vi "2022_day07.vi"() -> ()   [LabVIEW 2021]
uses:
  3baf8011-b907-4a24-9a6c-8a8b08bbcfa0.vi
  <vilib>/Comparison/Less/Less Functor/Less Functor.lvclass
panel:
  out "Task 2":i32
  out "Total Used Space":i32
  out "Task 1":i32
  in  "Switch":bool caption="Ex. Data  vs.  User Data"
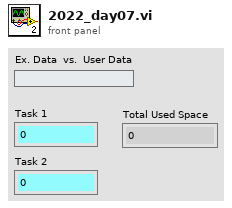
[diagram p1: front panel]
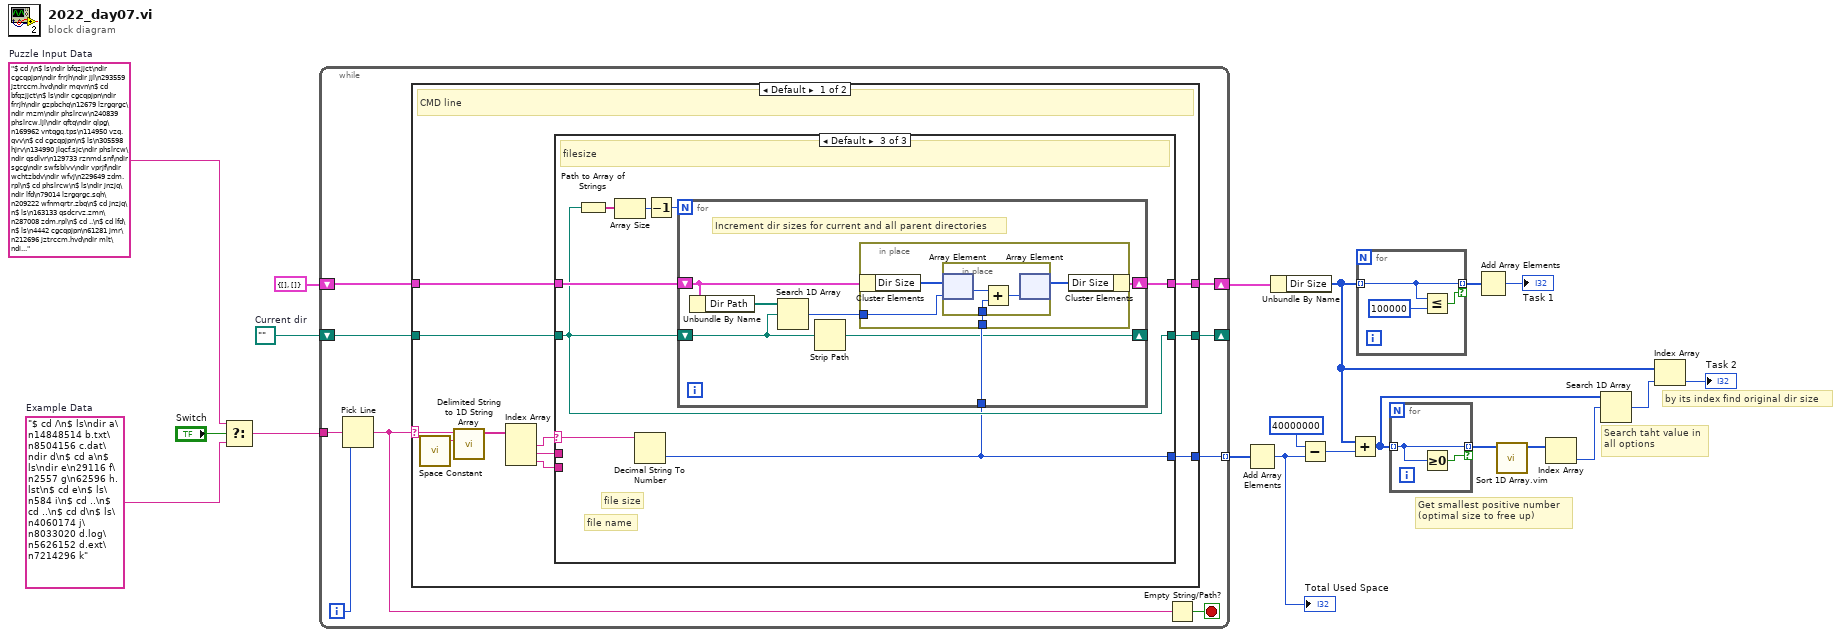
[diagram p0: block diagram]
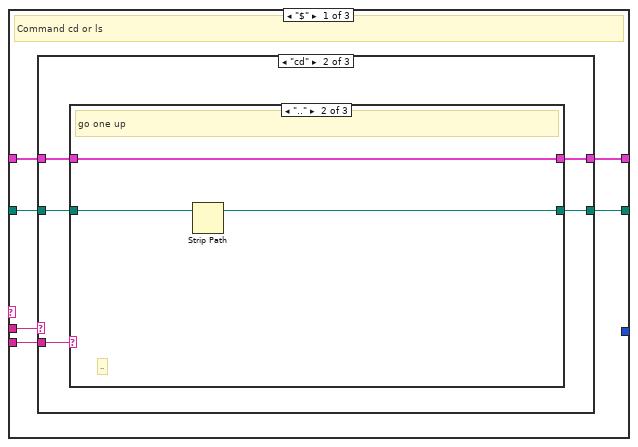
[diagram p2: hidden frame]
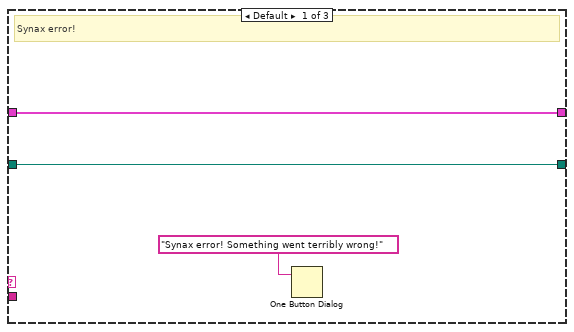
[diagram p3: hidden frame]
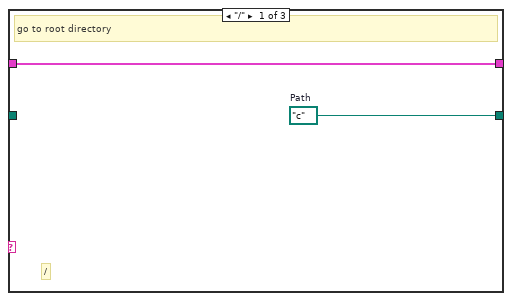
[diagram p4: hidden frame]
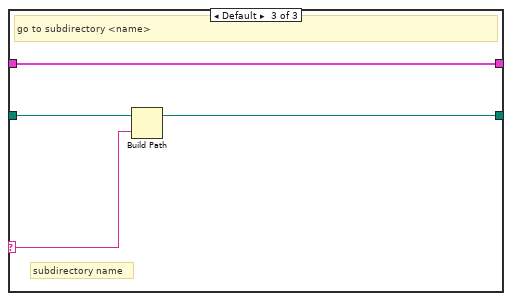
[diagram p5: hidden frame]
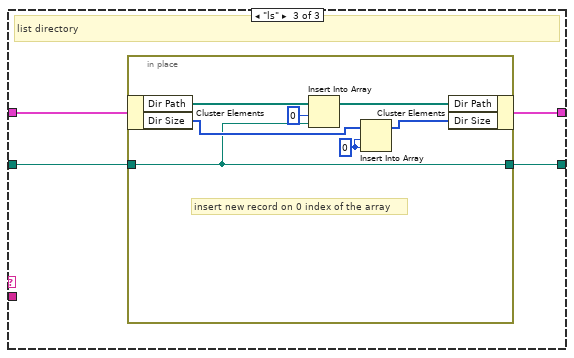
[diagram p6: hidden frame]
diagram:
  w15 = path ""  # Current dir
  w19 = "$ cd /\n$ ls\ndir bfqzjjct\ndir cgcqpjpn\ndir frrjh\ndir jjl\n293559 jztrccm.hvd\ndir mqvn\n$ cd bfqzjjct\n$ ls\ndir cgcqpjpn\ndir frrjh\ndir gzpbchq\n12679 lzrgqrgc\ndir mzm\ndir phslrcw\n240839 phslrcw.ljl\ndir qftq\ndir qlpg\n169962 vntqgq.tps\n114950 vzq.qvv\n$ cd cgcqpjpn\n$ ls\n305598 hjrv\n134990 jlqcf.sjc\ndir phslrcw\ndir qsdlvr\n129733 rznmd.snf\ndir sgcg\ndir swfsblvv\ndir vprjf\ndir wchtzbdv\ndir wfvj\n229649 zdm.rpl\n$ cd phslrcw\n$ ls\ndir jnzjq\ndir lfd\n79014 lzrgqrgc.sqh\n209222 wfnmqrtr.zbq\n$ cd jnzjq\n$ ls\n163133 qsdcrvz.zmn\n287008 zdm.rpl\n$ cd ..\n$ cd lfd\n$ ls\n4442 cgcqpjpn\n61281 jmr\n212696 jztrccm.hvd\ndir mlt\ndir qsdlvr\n$ cd mlt\n$ ls\n183050 zdm.rpl\n$ cd ..\n$ cd qsdlvr\n$ ls\ndir nzjfwdt\ndir qsdlvr\n$ cd nzjfwdt\n$ ls\n49044 jdqz.bqd\n$ cd ..\n$ cd qsdlvr\n$ ls\n13838 fpfmhq.rbp\n$ cd ..\n$ cd ..\n$ cd ..\n$ cd ..\n$ cd qsdlvr\n$ ls\n167042 jdqz.bqd\n132914 lzrgqrgc\n$ cd ..\n$ cd sgcg\n$ ls\ndir bjwzfr\n111567 jdqz.bqd\n33253 jztrccm.hvd\n75760 qsdlvr\n$ cd bjwzfr\n$ ls\n268763 npjd.glz\ndir phslrcw\n121486 vbfsrwf.mbc\ndir vtwtmnvl\n$ cd phslrcw\n$ ls\n114641 cgsrlq\n235130 npjd.glz\n$ cd ..\n$ cd vtwtmnvl\n$ ls\n7771 hnrpgsn\n290862 rtrljz.vbf\n220102 rztn.vqq\n$ cd ..\n$ cd ..\n$ cd ..\n$ cd swfsblvv\n$ ls\n231282 vclmcf.vpq\n16727 vjhmb.ftn\n$ cd ..\n$ cd vprjf\n$ ls\ndir fppsf\n56173 npjd.glz\ndir phslrcw\ndir pwjdcdff\ndir qsdlvr\ndir qvh\ndir sbmtlz\n$ cd fppsf\n$ ls\ndir hltnf\ndir qrmggjs\ndir qsdlvr\n$ cd hltnf\n$ ls\n201448 npjd.glz\n23616 zdm.rpl\n$ cd ..\n$ cd qrmggjs\n$ ls\ndir blhwqwd\ndir szf\n$ cd blhwqwd\n$ ls\n142887 vzq.qvv\n$ cd ..\n$ cd szf\n$ ls\n225491 tvsf.tpv\n$ cd ..\n$ cd ..\n$ cd qsdlvr\n$ ls\n92209 brmrwznr\ndir frrjh\n212979 qsdlvr.bwh\ndir vpvnb\n$ cd frrjh\n$ ls\n143811 qvwmpj.gnc\n$ cd ..\n$ cd vpvnb\n$ ls\ndir wwsw\n$ cd wwsw\n$ ls\n13671 qsdlvr\n$ cd ..\n$ cd ..\n$ cd ..\n$ cd ..\n$ cd phslrcw\n$ ls\ndir bpfhc\ndir fjvgwbj\n127950 hjngrw.rtr\n37045 lfpjb.ftz\ndir qsn\n$ cd bpfhc\n$ ls\n232351 frrjh.szf\n14824 jztrccm.hvd\n162270 vzq.qvv\n$ cd ..\n$ cd fjvgwbj\n$ ls\ndir cgcqpjpn\n4290 jrfsmghw.vqr\ndir lqnpdd\n$ cd cgcqpjpn\n$ ls\n208104 btrcq.vpn\n149676 bwvp.jlf\n76056 gvvrvqdf.zdc\n272686 pqhtjpv\ndir zjntbw\n$ cd zjntbw\n$ ls\n140092 jdqz.bqd\n$ cd ..\n$ cd ..\n$ cd lqnpdd\n$ ls\ndir brf\n197899 jdqz.bqd\ndir phslrcw\n236823 qcvgnlv.ngn\ndir szrfcwtw\n88974 vzq.qvv\n$ cd brf\n$ ls\n112059 jdqz.bqd\n217412 vzq.qvv\n$ cd ..\n$ cd phslrcw\n$ ls\n84285 jnzf\n282660 zdm.rpl\n$ cd ..\n$ cd szrfcwtw\n$ ls\n84415 gcp\n163787 wffb.wbq\n$ cd ..\n$ cd ..\n$ cd ..\n$ cd qsn\n$ ls\n139676 zdm.rpl\n$ cd ..\n$ cd ..\n$ cd pwjdcdff\n$ ls\ndir cgcqpjpn\n54163 lzrgqrgc\ndir qsdlvr\n51246 qsdlvr.cmq\n5082 rvmv.tqj\n112712 vzq.qvv\n$ cd cgcqpjpn\n$ ls\n92895 dmf.bsv\ndir lhqzc\n$ cd lhqzc\n$ ls\n13443 hwlsmmjn.wpj\n232141 tlsn\n$ cd ..\n$ cd ..\n$ cd qsdlvr\n$ ls\n216144 dghbz.lnl\n241311 jztrccm.hvd\n$ cd ..\n$ cd ..\n$ cd qsdlvr\n$ ls\n109764 qsdlvr.tbj\n$ cd ..\n$ cd qvh\n$ ls\ndir frrjh\n51428 hdtmm.zzl\n$ cd frrjh\n$ ls\n271661 brff.mgp\n$ cd ..\n$ cd ..\n$ cd sbmtlz\n$ ls\n277255 jztrccm.hvd\n$ cd ..\n$ cd ..\n$ cd wchtzbdv\n$ ls\n198310 cgcqpjpn\n300478 fcfvgpdr.lzv\n145860 jdqz.bqd\n20145 mggg\n$ cd ..\n$ cd wfvj\n$ ls\n270522 phslrcw.mwt\n213919 tczvr\n19226 zdm.rpl\n$ cd ..\n$ cd ..\n$ cd frrjh\n$ ls\ndir cgcqpjpn\n246391 hnc.bzl\ndir lzrgqrgc\ndir mnrbzwr\n239337 npjd.glz\ndir qsdlvr\n$ cd cgcqpjpn\n$ ls\n2423 pflhrgjg.gch\n$ cd ..\n$ cd lzrgqrgc\n$ ls\n265708 vzq.qvv\n107406 zwnjb\n$ cd ..\n$ cd mnrbzwr\n$ ls\n287289 jgs.bdb\n$ cd ..\n$ cd qsdlvr\n$ ls\ndir qsdlvr\n$ cd qsdlvr\n$ ls\n71204 gnfz\n$ cd ..\n$ cd ..\n$ cd ..\n$ cd gzpbchq\n$ ls\ndir cmqgph\ndir fwf\n146975 jztrccm.hvd\n284515 lzrgqrgc.qsf\n27455 qbsbvscc\n$ cd cmqgph\n$ ls\n177740 zdm.rpl\n$ cd ..\n$ cd fwf\n$ ls\n210658 dnmvdgwn.wzt\n22013 rqcspw.qmf\n244013 zdm.rpl\n$ cd ..\n$ cd ..\n$ cd mzm\n$ ls\n262805 gnfsbdcd.tvp\n$ cd ..\n$ cd phslrcw\n$ ls\n74949 wncqjc.tzd\n$ cd ..\n$ cd qftq\n$ ls\ndir jrds\n$ cd jrds\n$ ls\ndir dvht\ndir qsdlvr\n$ cd dvht\n$ ls\n57354 phslrcw\n57174 qsdlvr.ftm\n$ cd ..\n$ cd qsdlvr\n$ ls\n132030 fbsmfspp\n$ cd ..\n$ cd ..\n$ cd ..\n$ cd qlpg\n$ ls\ndir cgcqpjpn\ndir frrjh\ndir jjsfmg\n186178 jmvcvw\ndir qgjhlnmf\n100234 qltp.vdr\ndir tbwt\ndir vjjvfbdw\ndir wjz\n162428 zlbnsg\n$ cd cgcqpjpn\n$ ls\ndir gvmgcftp\ndir hsgvgc\ndir nps\ndir phslrcw\ndir scdglb\n$ cd gvmgcftp\n$ ls\n31869 dsddwbbp\ndir fbsrjgzj\n53280 tzn.fvp\n$ cd fbsrjgzj\n$ ls\n89267 qsdlvr.lhs\n$ cd ..\n$ cd ..\n$ cd hsgvgc\n$ ls\ndir lzrgqrgc\n210774 wpspf.vrd\n$ cd lzrgqrgc\n$ ls\n289086 gfhwwslq.tlz\n$ cd ..\n$ cd ..\n$ cd nps\n$ ls\n74713 fnqzcr\ndir srjvfq\n94736 wbrcn.nng\ndir wmddln\ndir zsgnrmcc\n$ cd srjvfq\n$ ls\ndir grqft\ndir pjnjlf\n254618 wmfnmfrc.wng\n$ cd grqft\n$ ls\n3742 zmpzwh.nvz\n$ cd ..\n$ cd pjnjlf\n$ ls\ndir mlrsrs\n$ cd mlrsrs\n$ ls\n167149 jztrccm.hvd\n$ cd ..\n$ cd ..\n$ cd ..\n$ cd wmddln\n$ ls\n222831 cgcqpjpn.dcv\n140188 gsvngqp\n174466 sfngrqgj.gvz\n$ cd ..\n$ cd zsgnrmcc\n$ ls\n143043 vzq.qvv\n$ cd ..\n$ cd ..\n$ cd phslrcw\n$ ls\ndir cdfsrvnc\n103523 hzsjc\n239089 jvwdjbq\n229835 npjd.glz\n189778 wwcccwmb.bdp\n$ cd cdfsrvnc\n$ ls\ndir vzsvcnlz\n$ cd vzsvcnlz\n$ ls\ndir wwn\n$ cd wwn\n$ ls\n60279 frngbwm.wwf\n$ cd ..\n$ cd ..\n$ cd ..\n$ cd ..\n$ cd scdglb\n$ ls\n176557 vzq.qvv\n$ cd ..\n$ cd ..\n$ cd frrjh\n$ ls\n130811 jdqz.bqd\n$ cd ..\n$ cd jjsfmg\n$ ls\ndir nffq\n22842 vzt.nwh\n$ cd nffq\n$ ls\ndir wmq\n$ cd wmq\n$ ls\n196322 jztrccm.hvd\n$ cd ..\n$ cd ..\n$ cd ..\n$ cd qgjhlnmf\n$ ls\ndir jhqqjt\ndir phslrcw\n246296 pzvmcq\n219308 tlhqgtcl.twb\ndir vfgb\n300258 zdm.rpl\n221663 zsqh.dph\n$ cd jhqqjt\n$ ls\n90068 fctpjdlm.ggg\ndir frrjh\ndir ngmzbqb\ndir phslrcw\n64341 qsdlvr.pnq\ndir vlgpcg\n$ cd frrjh\n$ ls\n49247 qrrhdhld.sjr\n$ cd ..\n$ cd ngmzbqb\n$ ls\n247800 cgcqpjpn.wgv\n$ cd ..\n$ cd phslrcw\n$ ls\ndir qsdlvr\ndir vjrrrm\n$ cd qsdlvr\n$ ls\n255302 ddvc\n182817 dzd.trp\n$ cd ..\n$ cd vjrrrm\n$ ls\n38983 hjbsqd.pdl\n$ cd ..\n$ cd ..\n$ cd vlgpcg\n$ ls\ndir frrjh\n83387 jztrccm.hvd\n$ cd frrjh\n$ ls\ndir rmlc\n$ cd rmlc\n$ ls\n273584 jztrccm.hvd\n$ cd ..\n$ cd ..\n$ cd ..\n$ cd ..\n$ cd phslrcw\n$ ls\n96286 jztrccm.hvd\n224425 npjd.glz\n$ cd ..\n$ cd vfgb\n$ ls\ndir fgl\ndir fllsgwjt\ndir frrjh\ndir qsdlvr\n$ cd fgl\n$ ls\n61972 lzrgqrgc.qrs\n$ cd ..\n$ cd fllsgwjt\n$ ls\ndir fqchdcpd\n214477 zcr.spz\n$ cd fqchdcpd\n$ ls\n156000 jccqlw.twl\n$ cd ..\n$ cd ..\n$ cd frrjh\n$ ls\n210987 zdm.rpl\n$ cd ..\n$ cd qsdlvr\n$ ls\ndir phslrcw\ndir znnsfvz\n$ cd phslrcw\n$ ls\n214655 ddw\n$ cd ..\n$ cd znnsfvz\n$ ls\n126028 zpq.bgs\n$ cd ..\n$ cd ..\n$ cd ..\n$ cd ..\n$ cd tbwt\n$ ls\ndir ltjjhr\n$ cd ltjjhr\n$ ls\n158069 vplwrz.rzp\n$ cd ..\n$ cd ..\n$ cd vjjvfbdw\n$ ls\n277114 fmndb.rth\n241524 frrjh\n212152 frrjh.dlq\n61370 jztrccm.hvd\ndir srvqm\n237264 znt\n$ cd srvqm\n$ ls\ndir fbzmddc\n61958 jdqz.bqd\ndir phslrcw\n173063 vwvmhwzn.tvg\n$ cd fbzmddc\n$ ls\ndir ccvtbpzw\n201647 lzrgqrgc.sjs\n192449 rhfgcgz\n224557 sbcpcbpd\n$ cd ccvtbpzw\n$ ls\ndir phslrcw\ndir prpllzcn\n$ cd phslrcw\n$ ls\n290780 lbl.qmm\n$ cd ..\n$ cd prpllzcn\n$ ls\n242024 bhq\n118347 frrjh.tsz\ndir hcqs\n$ cd hcqs\n$ ls\n104706 csnllvcf\n270940 npjd.glz\n$ cd ..\n$ cd ..\n$ cd ..\n$ cd ..\n$ cd phslrcw\n$ ls\n244909 czfjsrns.fdm\ndir frrjh\n68252 lzrgqrgc\n146640 npjd.glz\n290259 pbzpthgs.bgf\n99657 rmfpfmd\ndir zllf\n$ cd frrjh\n$ ls\ndir cgcqpjpn\n65295 jdqz.bqd\ndir phslrcw\n$ cd cgcqpjpn\n$ ls\ndir mwfwrd\n$ cd mwfwrd\n$ ls\n26481 sngtgc\ndir zfzddl\n$ cd zfzddl\n$ ls\n47854 fzfdrmbb.ngm\n$ cd ..\n$ cd ..\n$ cd ..\n$ cd phslrcw\n$ ls\n251021 fwfpd.vrt\n230149 fwjznjtz\n140480 gbsmhj\n112221 lzrgqrgc.gcr\n139564 npjd.glz\ndir pvmvm\ndir tpzr\n$ cd pvmvm\n$ ls\n73785 tnbgmgt.wqg\n$ cd ..\n$ cd tpzr\n$ ls\n16759 tmcmp\n$ cd ..\n$ cd ..\n$ cd ..\n$ cd zllf\n$ ls\n281402 dzrsnzh.smb\n$ cd ..\n$ cd ..\n$ cd ..\n$ cd ..\n$ cd wjz\n$ ls\n266826 cgcqpjpn.spr\ndir frvbfjj\n111126 jdqz.bqd\n257951 pbn.gdc\ndir vjs\ndir zrnvnb\n$ cd frvbfjj\n$ ls\n257181 glfdplrm\n$ cd ..\n$ cd vjs\n$ ls\ndir jmpbwhtj\n159996 lzrgqrgc.zcb\n192135 phw\ndir tdfz\ndir wtm\n$ cd jmpbwhtj\n$ ls\ndir fln\ndir frrjh\ndir nrtcmj\n$ cd fln\n$ ls\n284574 frrjh.scb\n$ cd ..\n$ cd frrjh\n$ ls\n10020 npjd.glz\n295395 vzq.qvv\n$ cd ..\n$ cd nrtcmj\n$ ls\ndir htvm\n$ cd htvm\n$ ls\ndir lwh\n$ cd lwh\n$ ls\n162494 npjd.glz\n$ cd ..\n$ cd ..\n$ cd ..\n$ cd ..\n$ cd tdfz\n$ ls\ndir gtvlbhhw\ndir hvssbj\ndir phslrcw\n$ cd gtvlbhhw\n$ ls\n172627 sjvcfz\ndir tfnhsrc\n76460 vvgcv\n$ cd tfnhsrc\n$ ls\ndir hjrjmrwc\n$ cd hjrjmrwc\n$ ls\n41459 jztrccm.hvd\n$ cd ..\n$ cd ..\n$ cd ..\n$ cd hvssbj\n$ ls\n64052 phslrcw\n$ cd ..\n$ cd phslrcw\n$ ls\ndir wtdpf\ndir zctdqwbc\n$ cd wtdpf\n$ ls\n75802 jztrccm.hvd\n$ cd ..\n$ cd zctdqwbc\n$ ls\n127648 vqzcf.wbl\n$ cd ..\n$ cd ..\n$ cd ..\n$ cd wtm\n$ ls\n265433 jztrccm.hvd\n20952 mplbrzlp\n123701 nwr.tjg\n58492 qsdlvr.qzq\n$ cd ..\n$ cd ..\n$ cd zrnvnb\n$ ls\n228205 ghllsc.fqn\n$ cd ..\n$ cd ..\n$ cd ..\n$ cd ..\n$ cd cgcqpjpn\n$ ls\ndir cmnsbsqp\ndir hzsn\n221975 jdqz.bqd\n177439 jztrccm.hvd\ndir mqjrcw\ndir tdp\n211065 zdm.rpl\n$ cd cmnsbsqp\n$ ls\n282903 qzlc\n$ cd ..\n$ cd hzsn\n$ ls\n221345 wtdnp.grd\n$ cd ..\n$ cd mqjrcw\n$ ls\n156244 gznmpr.dlr\n45213 hdb.fjb\n202993 pdt\ndir znvdz\n$ cd znvdz\n$ ls\n183973 jztrccm.hvd\n$ cd ..\n$ cd ..\n$ cd tdp\n$ ls\n68564 nmntwl\n259117 vzq.qvv\n$ cd ..\n$ cd ..\n$ cd frrjh\n$ ls\n276034 lzrgqrgc.fgq\ndir psqczq\ndir qsdlvr\ndir snrw\n$ cd psqczq\n$ ls\n158415 jdqz.bqd\n127684 lhctqnnz.hgn\n123191 phslrcw.prl\ndir wrftp\n$ cd wrftp\n$ ls\n234327 qdbbl.czd\n$ cd ..\n$ cd ..\n$ cd qsdlvr\n$ ls\n179591 chbns.sqf\n88327 jdqz.bqd\ndir mrf\n$ cd mrf\n$ ls\n229849 phslrcw.rdr\n$ cd ..\n$ cd ..\n$ cd snrw\n$ ls\ndir cbvr\ndir lbbrtc\n134786 lzrgqrgc.vrt\n131987 vzq.qvv\n$ cd cbvr\n$ ls\n120330 htmgqj.nbq\n162963 lzrgqrgc.rwq\n$ cd ..\n$ cd lbbrtc\n$ ls\ndir tnqdj\n$ cd tnqdj\n$ ls\n72261 lhqnwns.nhj\n235520 qsdlvr.dtr\n$ cd ..\n$ cd ..\n$ cd ..\n$ cd ..\n$ cd jjl\n$ ls\ndir fcfpptw\ndir frrjh\ndir gmdwgs\n221258 jdqz.bqd\ndir lzrgqrgc\ndir mwnmjjj\n297139 smjtpl.zzs\n$ cd fcfpptw\n$ ls\n167264 frrjh\n101587 hsmhhc.lvb\n$ cd ..\n$ cd frrjh\n$ ls\n268280 jztrccm.hvd\n127939 nbqgvd\n247875 nmnrsqq\ndir phslrcw\ndir rmgwbq\n288264 znrrdmw\n$ cd phslrcw\n$ ls\ndir cgcqpjpn\ndir nbwjw\n$ cd cgcqpjpn\n$ ls\n249503 phslrcw.dmf\n$ cd ..\n$ cd nbwjw\n$ ls\ndir phslrcw\n$ cd phslrcw\n$ ls\n193336 sqpgwtgp.fpb\n$ cd ..\n$ cd ..\n$ cd ..\n$ cd rmgwbq\n$ ls\n90116 jztrccm.hvd\n303005 phslrcw\n$ cd ..\n$ cd ..\n$ cd gmdwgs\n$ ls\ndir lzrgqrgc\ndir mwrj\ndir mzqn\n104570 qsqqbfg.njt\ndir zmj\n$ cd lzrgqrgc\n$ ls\ndir cmn\ndir qsdlvr\ndir rtz\n$ cd cmn\n$ ls\n20043 bgm.tvn\n41301 hqdl.rnr\n32026 tsmmr.bfl\n$ cd ..\n$ cd qsdlvr\n$ ls\ndir dcsdmqt\n$ cd dcsdmqt\n$ ls\n107938 zdm.rpl\n$ cd ..\n$ cd ..\n$ cd rtz\n$ ls\n308963 jbwvpjvj.fgn\n31573 jdqz.bqd\n97775 phslrcw\ndir qsdlvr\n225929 wwznl.bpd\n$ cd qsdlvr\n$ ls\n52056 bddqnlmg.hjm\n236614 qsdlvr.vcz\n$ cd ..\n$ cd ..\n$ cd ..\n$ cd mwrj\n$ ls\ndir dfsm\ndir mtfqs\n$ cd dfsm\n$ ls\n32797 jztrccm.hvd\ndir mthjq\n241875 vzq.qvv\n$ cd mthjq\n$ ls\n147247 zdm.rpl\n$ cd ..\n$ cd ..\n$ cd mtfqs\n$ ls\ndir crpfs\ndir phslrcw\n$ cd crpfs\n$ ls\n24073 jdqz.bqd\n269270 jztrccm.hvd\n89807 lzrgqrgc.ddj\n$ cd ..\n$ cd phslrcw\n$ ls\n124727 cgcqpjpn.zfz\ndir gttptlwj\ndir phslrcw\ndir qsdlvr\n$ cd gttptlwj\n$ ls\n295546 frrjh.tmq\n$ cd ..\n$ cd phslrcw\n$ ls\n234122 zdm.rpl\n$ cd ..\n$ cd qsdlvr\n$ ls\n131491 zdm.rpl\n$ cd ..\n$ cd ..\n$ cd ..\n$ cd ..\n$ cd mzqn\n$ ls\n16352 qjllmbh.jfm\n36853 zdm.rpl\n$ cd ..\n$ cd zmj\n$ ls\ndir dvrwbrbt\ndir frrjh\n217060 mftczjfs.zch\ndir znhsrsfb\n$ cd dvrwbrbt\n$ ls\ndir lzssrrq\n$ cd lzssrrq\n$ ls\ndir qsdlvr\n$ cd qsdlvr\n$ ls\n108975 npjd.glz\n$ cd ..\n$ cd ..\n$ cd ..\n$ cd frrjh\n$ ls\ndir phslrcw\ndir zjstpvl\n$ cd phslrcw\n$ ls\n244682 pgn.jqm\n$ cd ..\n$ cd zjstpvl\n$ ls\n300736 bsw.wzn\n102742 jdqz.bqd\n$ cd ..\n$ cd ..\n$ cd znhsrsfb\n$ ls\n121093 qsdlvr\n$ cd ..\n$ cd ..\n$ cd ..\n$ cd lzrgqrgc\n$ ls\n50942 jdqz.bqd\n26201 ljqgqqrr\n71462 lrrfvs.ghl\n274208 tqhcl.hcl\n$ cd ..\n$ cd mwnmjjj\n$ ls\n184865 mzwmp.jbw\n68016 thbh.nbg\n$ cd ..\n$ cd ..\n$ cd mqvn\n$ ls\n287623 spfzctll\n"  # Puzzle Input Data
  w18 = "$ cd /\n$ ls\ndir a\n14848514 b.txt\n8504156 c.dat\ndir d\n$ cd a\n$ ls\ndir e\n29116 f\n2557 g\n62596 h.lst\n$ cd e\n$ ls\n584 i\n$ cd ..\n$ cd ..\n$ cd d\n$ ls\n4060174 j\n8033020 d.log\n5626152 d.ext\n7214296 k"  # Example Data
  # "by its index find original dir size"
  # "Search taht value in\nall options"
  # "Get smallest positive number\n(optimal size to free up)"
  n1 = Select(t=w19, s="Switch", f=w18) -> (s? t:f=w17:string)
  n2 = while {
    tunnel: w17 -> [w29]
    shift-right: [w24] -> _
    shift-left: w15 -> [w25]
    shift-right: [w23] -> w14
    shift-left: cluster{"Dir Path":path[], "Dir Size":i32[]} {"Dir Path"=[], "Dir Size"=[]} -> [w22]
    tunnel: [w21] -> w11 mode=indexing
    i -> [w26]
    stop <- w28 stop-if-true
    n3 = Pick Line(multi-line string=w29, line index=w26) -> (output string=w27:string)  [unwired: 1 in]
    n4 = case shown="Default" w27 {
      selector: w27 -> [w40 _]
      tunnel: w25 -> [w37 w100]
      tunnel: [w36 w100] -> w24
      tunnel: [w35 w99] -> w23
      tunnel: w22 -> [w34 w99]
      tunnel: [w30 _] -> w21
      frame Default {
        # "CMD line"
        n5 = call <vilib>:"Space Constant.vi"() -> ("String"=w39:string)
        n6 = call <vilib>:"Delimited String to 1D String Array.vi"("delimiter"=w39, "delimited string"=w40) -> ("string array"=w32:string[])  [unwired: 9 in]
        n7 = Index Array(array=w32) -> (element #1=w38:string, element #2=w33:string, element #3=w31:string)  [unwired: 3 in]
        n8 = case shown="Default" w38 {
          selector: w38 -> [_ _ w84]
          tunnel: w37 -> [w44 w76 w81]
          tunnel: [w43 w76 w81] -> w36
          tunnel: [w46 w75 w82] -> w35
          tunnel: w34 -> [w45 w75 w83]
          tunnel: w33 -> [w42 _ _]
          tunnel: w31 -> [w41 _ _]
          tunnel: [_ _ w77] -> w30
          frame "$" {
            # "Command cd or ls"
            n9 = case shown="\"cd\"" w42 {
              tunnel: [w49 w53 w64] -> w46
              tunnel: w45 -> [w49 w52 w67]
              tunnel: w44 -> [w48 w51 w66]
              tunnel: [w48 w50 w65] -> w43
              tunnel: w41 -> [_ w54 _]
              frame Default {
                # "Synax error!"
                n10 = One Button Dialog(message="Synax error! Something went terribly wrong!") -> ()  [unwired: 1 in, 1 out]
              }
              frame "cd" {
                n11 = case shown="\"..\"" w54 {
                  selector: w54 -> [_ _ w61]
                  tunnel: [w56 w59 w63] -> w53
                  tunnel: w52 -> [w56 w59 w63]
                  tunnel: w51 -> [_ w57 w60]
                  tunnel: [w55 w58 w62] -> w50
                  frame "/" {
                    w55 = path "c:/"  # Path
                    # "/"
                    # "go to root directory"
                  }
                  frame ".." {
                    # ".."
                    # "go one up"
                    n12 = Strip Path(path=w57) -> (stripped path=w58:path)  [unwired: 1 out]
                  }
                  frame Default {
                    # "subdirectory name"
                    # "go to subdirectory <name>"
                    n13 = Build Path(base path=w60, name or relative path=w61) -> (appended path=w62:path)
                  }
                }
              }
              frame "ls" {
                # "list directory"
                n14 = in-place {
                  in-place-border: w66 -> [w70]
                  in-place-border: [w70] -> w65
                  w69 = 0 ("new element/subarray")
                  # "insert new record on 0 index of the array"
                  n15 = in-place-cluster #1(w67) -> ("Dir Path"=w74:path[], "Dir Size"=w72:i32[])
                  n16 = Insert Into Array(array=w74, index=0, new element=w70) -> (w73:path[])
                  n17 = Insert Into Array(array=w72, index=w69, new element=w69) -> (w71:i32[])
                  n18 = in-place-cluster #1("Dir Path"=w73, "Dir Size"=w71) -> (w64:cluster{"Dir Path":path[], "Dir Size":i32[]})
                }
              }
            }
          }
          frame "dir" {
            # "dir name - do nothing"
          }
          frame Default {
            # "file name"
            # "file size"
            # "filesize"
            n19 = Path to Array of Strings(0:w81) -> (2:w79:string[])  [unwired: 1 out]
            n20 = Array Size(array=w79) -> (size(s)=w80:i32)
            n21 = Decimal String To Number(string=w84) -> (number=w77:i32)  [unwired: 2 in, 1 out]
            n22 = Decrement(x=w80) -> (x-1=w78:i32)
            n23 = for {
              N: w78 -> [_]
              tunnel: w77 -> [w91]
              shift-right: [w86] -> _
              shift-left: w81 -> [w87]
              shift-right: [w90] -> w82
              shift-left: w83 -> [w89]
              # "Increment dir sizes for current and all parent directories"
              n24 = Unbundle By Name(w89) -> ("Dir Path"=w88:path[])
              n25 = Search 1D Array(1D array=w88, element=w87) -> (index of element=w85:i32)  [unwired: 1 in]
              n26 = Strip Path(path=w87) -> (stripped path=w86:path)  [unwired: 1 out]
              n27 = in-place {
                in-place-border: w91 -> [w93]
                in-place-border: w85 -> [w92]
                n28 = in-place-cluster #2(w89) -> ("Dir Size"=w95:i32[])
                n29 = in-place {
                  in-place-border: w93 -> [w98]
                  n30 = in-place-array #3(w95, w92) -> (w97:i32)
                  n31 = Add(x=w97, y=w98) -> (x+y=w96:i32)
                  n32 = in-place-array #3(w96) -> (w94:i32[])  [unwired: 1 out]
                }
                n33 = in-place-cluster #2("Dir Size"=w94) -> (w90:cluster{"Dir Path":path[], "Dir Size":i32[]})
              }
            }
          }
        }
      }
      frame "" {
        # "End of file"
      }
    }
    n34 = Empty String/Path?(string/path=w27) -> (empty?=w28:bool)
  }
  n35 = Add Array Elements(numeric array=w11) -> (sum=w9:i32)
  "Total Used Space" <- w9
  n36 = Unbundle By Name(w14) -> ("Dir Size"=w2:i32[])
  n37 = Subtract(x=40000000 ("y"), y=w9) -> (x-y=w8:i32)
  n38 = Add(x=w2, y=w8) -> (x+y=w4:i32[])
  n39 = for {
    tunnel: w2 -> [w103] mode=indexing
    tunnel: [w103] -> w13 mode=indexing if=w101
    n40 = Less Or Equal?(x=w103, y=100000) -> (x <= y?=w101:bool)
  }
  n41 = for {
    tunnel: w4 -> [w105] mode=indexing
    tunnel: [w105] -> w7 mode=indexing if=w104
    n42 = Greater Or Equal To 0?(x=w105) -> (x >= 0?=w104:bool)
  }
  n43 = Add Array Elements(numeric array=w13) -> (sum=→"Task 1":i32)
  n44 = call "Sort 1D Array.vim"("unsorted array"=w7) -> ("sorted array"=w6:i32[])  [unwired: 10 in]
  n45 = Index Array(array=w6) -> (element=w5:i32)  [unwired: 1 in]
  n46 = Search 1D Array(1D array=w4, element=w5) -> (index of element=w3:i32)  [unwired: 1 in]
  n47 = Index Array(array=w2, index=w3) -> (element=→"Task 2":i32)
